vi "Flatten Value.vi"(8 "Error In":errorcluster, 11 "Float In":refnum<class "Flt.lvclass">) -> (0 "Error Out":errorcluster, 1 "Value":string, 3 "Float Out":refnum<class "Flt.lvclass">)   [LabVIEW 2020, in "NI_VIAnCFGDataStructure.lvlib" / "Flt.lvclass"]
uses:
  <vilib>/addons/analyzer/VIAnCFGDataStructure/Data Types/Float/Flt.lvclass
  <vilib>/addons/analyzer/VIAnCFGDataStructure/Data Types/Float/Flt.lvclass/Flt.ctl
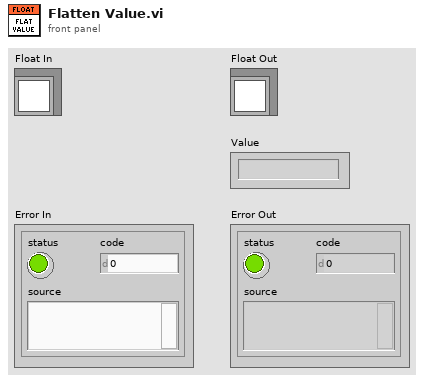
[diagram p1: front panel]
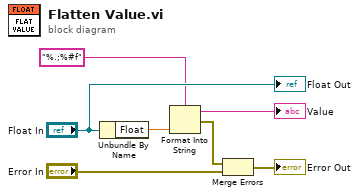
[diagram p0: block diagram]
diagram:
  n1 = Unbundle By Name("Float In") -> ("Float"=w2:dbl)
  n2 = Format Into String(format string="%.;%#f" ("initial string"), w2) -> (resulting string=→"Value":string, error out=w5:errorcluster)  [unwired: 2 in]
  n3 = Merge Errors(w5, "Error In") -> (→"Error Out":errorcluster)
  "Float Out" <- "Float In"
